vi "WPI_Gyro_ADXRS453_ParseSensorData.vi"(9 "Offset":dbl, 10 "Data":u8[](array[numeric])) -> (0 "Data Good":bool, 1 "Sequence":u8, 2 "Angular Rate (deg/sec)":dbl)   [LabVIEW 2017]
uses:
  <vilib>/Rock Robotics/WPI/Gyro/ADXRS453/WPI_Gyro_ADXRS453_Status.ctl
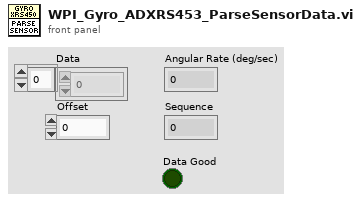
[diagram p1: front panel]
types:
  T1 = typedef "WPI_Gyro_ADXRS453_Status.ctl" = enum8{"Invalid", "Valid", "Self-Test", "Read/Write"}
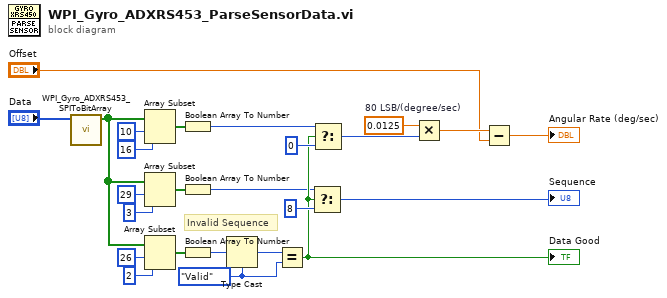
[diagram p0: block diagram]
diagram:
  w22 = 0.0125  # 80 LSB/(degree/sec)
  w15 = WPI_Gyro_ADXRS453_Status."Valid"
  # "Invalid Sequence"
  n1 = call <vilib>:"WPI_Gyro_ADXRS453_SPIToBitArray.vi"("SPI Byte Array (MSB first)"="Data") -> ("32-bit Boolean array"=w11:bool[])  [unwired: 10 in]
  n2 = Array Subset(array=w11, index=10, length=16) -> (w3:bool[])
  n3 = Array Subset(array=w11, index=29, length=3) -> (w8:bool[])
  n4 = Array Subset(array=w11, index=26, length=2) -> (w12:bool[])
  n5 = Boolean Array To Number(Boolean array=w3) -> (number=w16:i16)
  n6 = Boolean Array To Number(Boolean array=w8) -> (number=w17:u8)
  n7 = Boolean Array To Number(Boolean array=w12) -> (number=w13:u8)
  n8 = Type Cast(type=w15, x=w13) -> (*(type *) &x=w14:T1)
  n9 = Equal?(x=w14, y=w15) -> (x = y?=w18:bool)
  "Data Good" <- w18
  n10 = Select(t=w17, s=w18, f=u8 8) -> (s? t:f=→"Sequence":u8)
  n11 = Select(t=w16, s=w18, f=i16 0) -> (s? t:f=w23:i16)
  n12 = Multiply(x=w22, y=w23) -> (x*y=w25:dbl)
  n13 = Subtract(x=w25, y="Offset") -> (x-y=→"Angular Rate (deg/sec)":dbl)
